vi "Autonomous Independent.vi"() -> ()   [LabVIEW 2012]
doc: "This VI is called when autonomous begins, and will automatically be terminated when autonomous ends. You can carry out timed or sensor driven robot movement independently without needing to return to the caller."
uses:
  Robot Global Data.vi
  <vilib>/Rock Robotics/WPI/RobotDrive/WPI_RobotDriveArcadeDrive_Standard(NoSaturation).vi
panel:
  out "Shooter Tolerance":dbl
  out "Mode":u32
  out "Auton Mode":bool[](array[boolean])
  in  "Blank 2":i32=7
  in  "Blank 1":i32
  out "Driver Station":bool[](array[boolean])
  out "Auton RPM Used":dbl
  out "Auton Pitch Used":dbl
  in  "Auton RPM 2":dbl=4200.0
  in  "Auton Pitch 2":dbl=29.5
  out "Analog 1 (V)":dbl
  out "Autonomous Modes":T1(ring)
  out "Current Movement, for debugging":T2 {"Y Joystick Value" scale=1.0..-1.0; "X Joystick Value" scale=-1.0..1.0}
  in  "Array of robot movements":T3(array[cluster]) {"Y Joystick Value" scale=1.0..-1.0; "X Joystick Value" scale=-1.0..1.0}
  # "Palmetto: Auton RPM was 4200, Pitch was 29.5"
  # "WING"
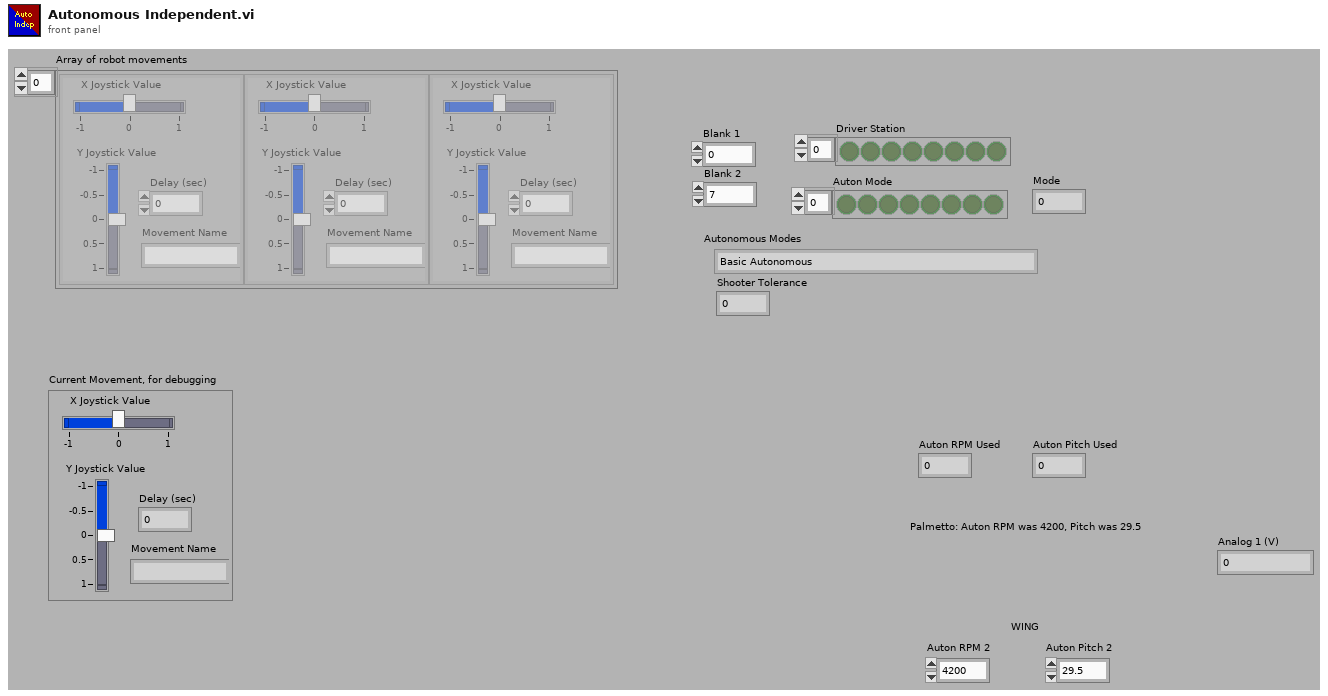
[diagram p1: front panel]
types:
  T1 = enum16{"Basic Autonomous", "Delayed Autonomous", "Shoot and Line Up With Protected Feeder Station", "Shoot and Line Up With Unprotected Feeder Station"}
  T2 = cluster{"X Joystick Value":dbl, "Y Joystick Value":dbl, "Delay (sec)":dbl, "Movement Name":string}
  T3 = cluster{"X Joystick Value":dbl, "Y Joystick Value":dbl, "Delay (sec)":dbl, "Movement Name":string}[]
  T4 = typedef "WPI_JoystickDevRef.ctl" = cluster{"Device":T5}
  T5 = typedef "WPI_JoystickDeviceEnum.ctl" = enum16{"USB 1", "USB 2", "USB 3", "USB 4", "Kinect 1", "Kinect 2"}
  T6 = cluster{"axis 1 (x)":dbl, "axis 2 (y)":dbl, "axis 3 (throttle)":dbl, "axis 4":dbl, "axis 5":dbl, "axis 6":dbl}
  T7 = typedef "WPI_RobotDriveDevRef.ctl" = cluster{"DevStatus":errorcluster, "Motors[]":T8[], "Square Inputs":bool, "Max Output":dbl, "Isochronous":bool}
  T8 = typedef "WPI_MotorControlDeviceRef.ctl" = cluster{"DeviceStatus":errorcluster, "Type":enum16{"PWM", "CAN"}, "PWM":cluster{"Digital Module":T9, "PWM Channel":T10, "DeadBand":T11}, "CAN":cluster{"Device Number":u8, "Control Mode":T12, "Semaphore":T13, "Max Vout":dbl}, "Invert":bool, "TransformRef":T14, "InvTransformRef":T14}
  T9 = typedef "FPGA_TypedefDigitalModule.ctl" = enum16{"Digital Module 1", "Digital Module 2"}
  T10 = typedef "FPGA_DIOPWMChannel.ctl" = enum8{"PWM 1", "PWM 2", "PWM 3", "PWM 4", "PWM 5", "PWM 6", "PWM 7", "PWM 8", "PWM 9", "PWM 10", "Invalid"}
  T11 = typedef "WPI_PWMDeadband.ctl" = cluster{"Name":string, "maxPositivePwm":i32, "minPositivePwm":i32, "centerPwm":i32, "maxNegativePwm":i32, "minNegativePwm":i32, "angularRange":u16}
  T12 = typedef "WPI_CANJaguar_ControlMode.ctl" = enum8{"Percent VBus", "Current", "Speed", "Position", "Voltage"}
  T13 = typedef "Semaphore RefNum" = refnum<k1>
  T14 = typedef "WPI_PWMTransform_ConPane.ctl" = refnum<vi>
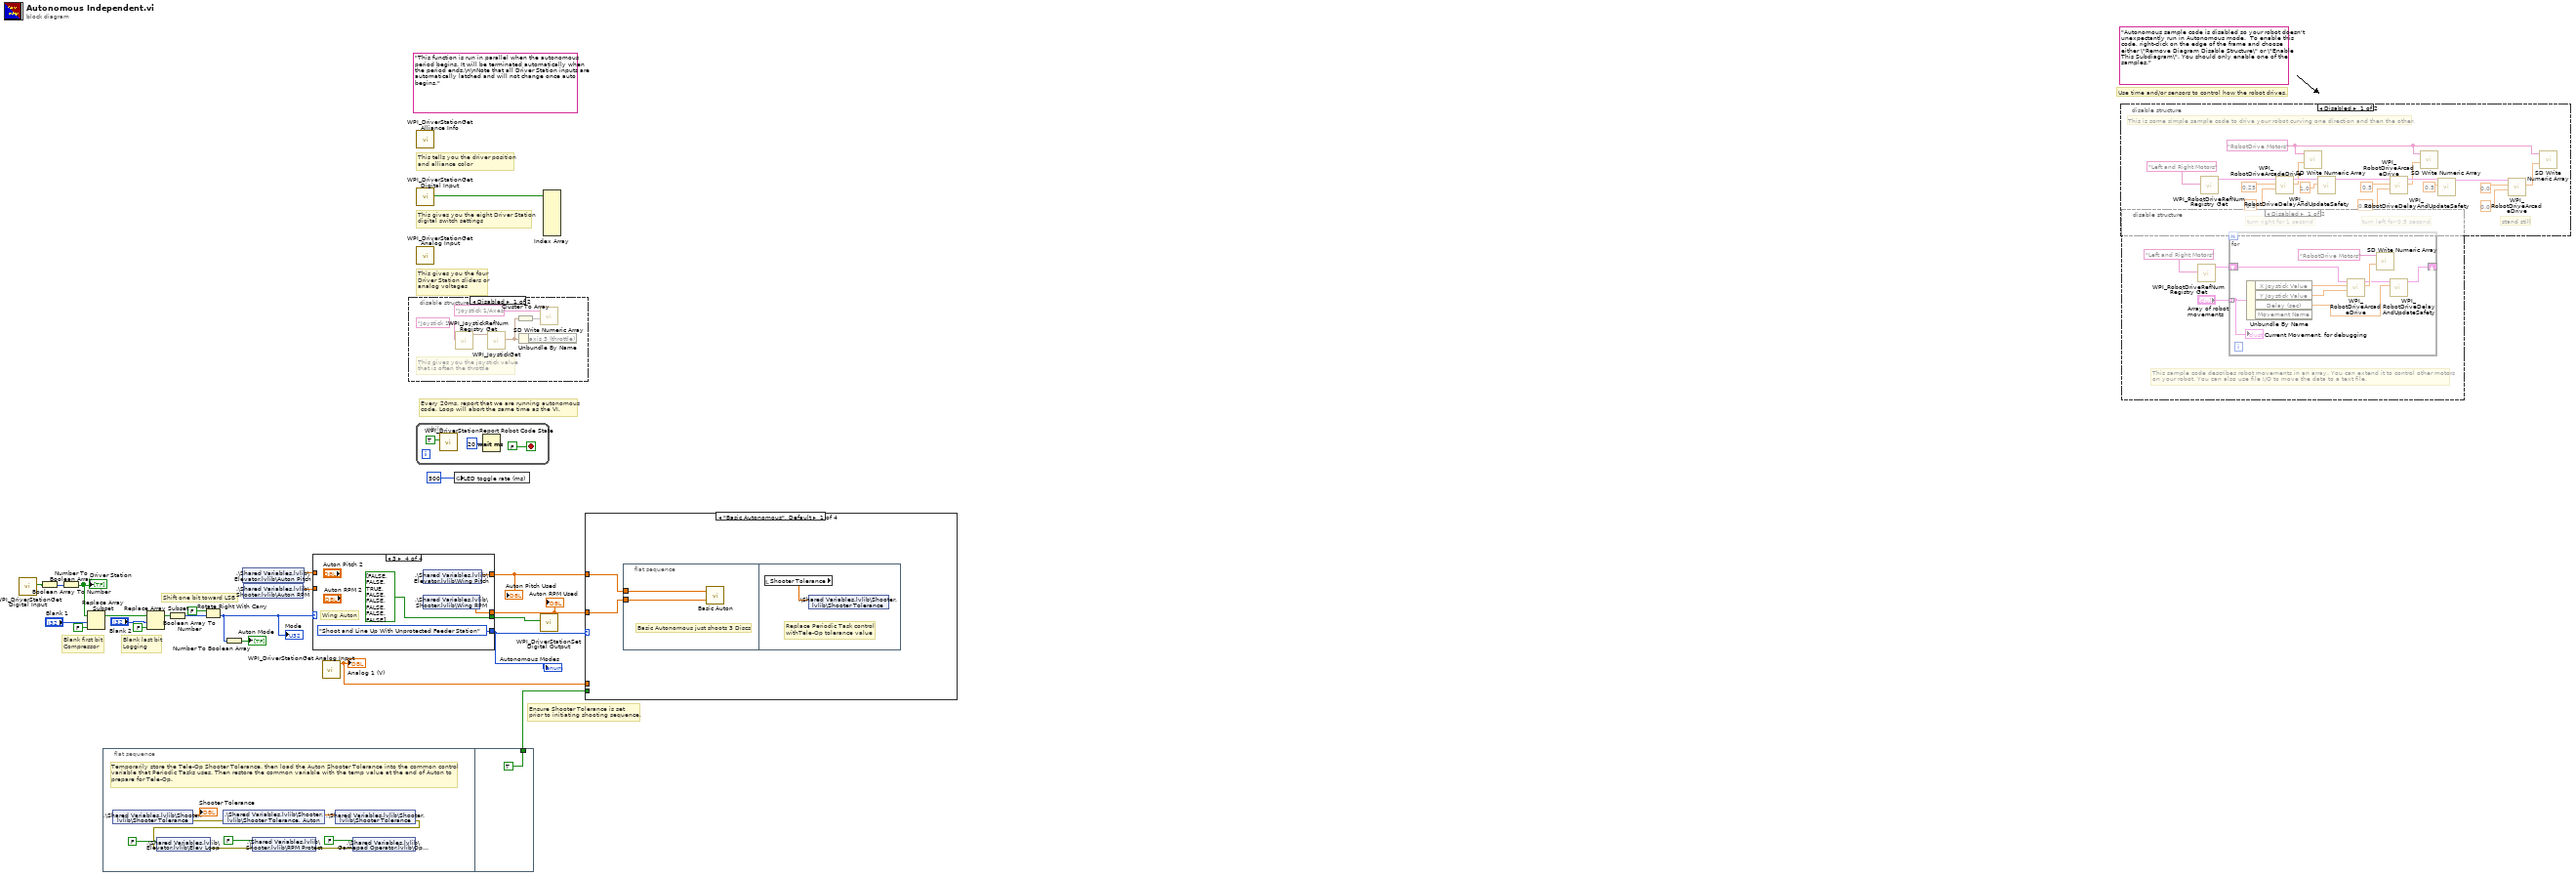
[diagram p0: block diagram]
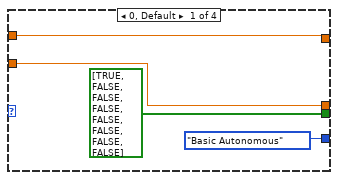
[diagram p3: hidden frame]
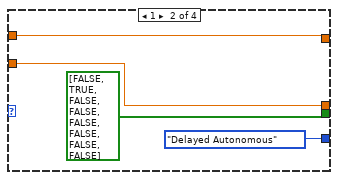
[diagram p4: hidden frame]
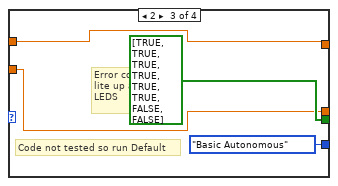
[diagram p5: hidden frame]
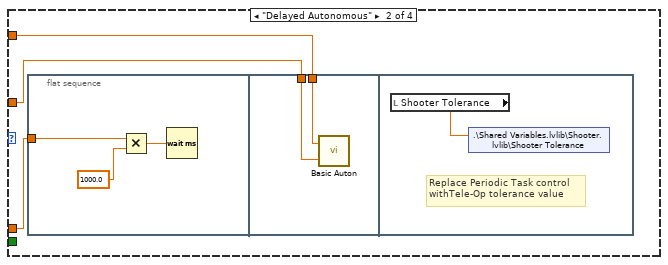
[diagram p6: hidden frame]
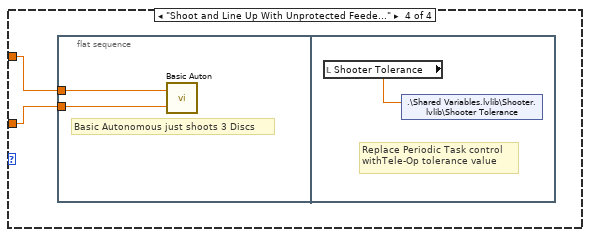
[diagram p8: hidden frame]
diagram:
  (unwired) "Autonomous sample code is disabled so your robot doesn't unexpectantly run in Autonomous mode.  To enable this code, right-click on the edge of the frame and choose either \"Remove Diagram Disable Structure\" or \"Enable This Subdiagram\". You should only enable one of the samples."
  (unwired) "This function is run in parallel when the autonomous period begins. It will be terminated automatically when the period ends.\n\nNote that all Driver Station inputs are automatically latched and will not change once auto begins."
  # "Ensure Shooter Tolerance is set\nprior to initiating shooting sequence."
  # "Shift one bit toward LSB"
  # "Blank last bit\nLogging"
  # "Blank first bit\nCompressor"
  # "Every 20ms, report that we are running autonomous\ncode. Loop will abort the same time as the VI."
  # "Use time and/or sensors to control how the robot drives."
  # "This tells you the driver position\nand alliance color"
  # "This gives you the eight Driver Station\ndigital switch settings"
  # "This gives you the four\nDriver Station sliders or\nanalog voltages"
  n1 = call <vilib>:"WPI_DriverStationGet Digital Input.vi"() -> ("Driver Station Digital Input (1-8)"=w19:bool[])  [unwired: 11 in]
  n2 = Boolean Array To Number(Boolean array=w19) -> (number=w5:u32)
  n3 = Number To Boolean Array(number=w5) -> (Boolean array=w15:bool[])
  "Driver Station" <- w15
  n4 = Replace Array Subset(array=w15, new element=FALSE ("new element/subarray"), index="Blank 1") -> (w10:bool[])
  n5 = flat-sequence {
    tunnel: [TRUE] -> w1
    frame #0 {
      # "Temporarily store the Tele-Op Shooter Tolerance, then load the Auton Shooter Tolerance into the common control \nvariable that Periodic Tasks uses. Then restore the common variable with the temp value at the end of Auton to \nprepare for Tele-Op."
      n6 = shared-variable ".\\Shared Variables.lvlib\\Shooter.lvlib\\Shooter Tolerance"() -> (→"Shooter Tolerance":dbl, error out=w27:errorcluster)  [unwired: 1 in]
      n7 = shared-variable ".\\Shared Variables.lvlib\\Shooter.lvlib\\Shooter Tolerance, Auton"(error in=w27) -> (w29:dbl)  [unwired: 1 out]
      n8 = shared-variable ".\\Shared Variables.lvlib\\Shooter.lvlib\\Shooter Tolerance"(w29) -> (error out=w26:errorcluster)  [unwired: 1 in]
      n9 = shared-variable ".\\Shared Variables.lvlib\\Elevator.lvlib\\Elev Loop"(FALSE ("ElevLoop"), error in=w26) -> (error out=w25:errorcluster)
      n10 = shared-variable ".\\Shared Variables.lvlib\\Shooter.lvlib\\RPM Protect"(FALSE ("collector_override"), error in=w25) -> (error out=w24:errorcluster)
      n11 = shared-variable ".\\Shared Variables.lvlib\\Gamepad Operator.lvlib\\Op Button 4"(FALSE ("Loading"), error in=w24) -> ()  [unwired: 1 out]
    }
    frame #1 {
    }
  }
  n12 = Replace Array Subset(array=w10, new element=FALSE ("new element/subarray"), index="Blank 2") -> (w9:bool[])
  n13 = Boolean Array To Number(Boolean array=w9) -> (number=w7:u32)
  n14 = Rotate Right With Carry(2:w7, 3:FALSE ("carry")) -> (0:w4:u32)  [unwired: 1 out]
  "Mode" <- w4
  n15 = Number To Boolean Array(number=w4) -> (Boolean array=→"Auton Mode":bool[])
  n16 = shared-variable ".\\Shared Variables.lvlib\\Elevator.lvlib\\Auton Pitch"() -> (w2:dbl)  [unwired: 1 in, 1 out]
  n17 = shared-variable ".\\Shared Variables.lvlib\\Shooter.lvlib\\Auton RPM"() -> (w3:dbl)  [unwired: 1 in, 1 out]
  n18 = case shown="3" w4 {
    tunnel: [T1."Basic Autonomous" ("Autonomous Modes") T1."Delayed Autonomous" ("Autonomous Modes") T1."Basic Autonomous" ("Autonomous Modes") T1."Shoot and Line Up With Unprotected Feeder Station" ("Autonomous Modes")] -> w21
    tunnel: [bool[] [TRUE, FALSE, FALSE, FALSE, FALSE, FALSE, FALSE, FALSE] ("Driver Station Digital Output (1-8)") bool[] [FALSE, TRUE, FALSE, FALSE, FALSE, FALSE, FALSE, FALSE] ("Driver Station Digital Output (1-8)") bool[] [TRUE, TRUE, TRUE, TRUE, TRUE, TRUE, FALSE, FALSE] ("Driver Station Digital Output (1-8)") bool[] [FALSE, FALSE, TRUE, FALSE, FALSE, FALSE, FALSE, FALSE] ("Driver Station Digital Output (1-8)")] -> w18
    tunnel: [w35 w39 w43 w47] -> w17
    tunnel: [w34 w38 w42 w46] -> w16
    tunnel: w2 -> [w35 w39 w43 _]
    tunnel: w3 -> [w34 w38 w42 _]
    frame 0, Default {
    }
    frame 1 {
    }
    frame 2 {
      # "Error cond\nlite up all\nLEDS"
      # "Code not tested so run Default"
    }
    frame 3 {
      # "Wing Auton"
      n19 = shared-variable ".\\Shared Variables.lvlib\\Elevator.lvlib\\Wing Pitch"() -> (w47:dbl)  [unwired: 1 in, 1 out]
      n20 = shared-variable ".\\Shared Variables.lvlib\\Shooter.lvlib\\Wing RPM"() -> (w46:dbl)  [unwired: 1 in, 1 out]
    }
  }
  "Autonomous Modes" <- w21
  "Auton Pitch Used" <- w17
  "Auton RPM Used" <- w16
  n21 = call <vilib>:"WPI_DriverStationGet Analog Input.vi"() -> ("Analog 1 (V)"=w20:dbl)  [unwired: 8 in, 3 out]
  "Analog 1 (V)" <- w20
  n22 = disable-structure shown="Disabled" {
    frame Disabled {
      # "This gives you the joystick value\nthat is often the throttle"
      n23 = call <vilib>:"WPI_JoystickRefNum Registry Get.vi"("refnum name"="Joystick 1") -> ("JoystickDevRef"=w53:T4)  [unwired: 1 in, 9 out]
      n24 = call <vilib>:"WPI_JoystickGet.vi"("JoystickDevRef"=w53) -> ("Axes"=w51:T6)  [unwired: 1 in, 5 out]
      n25 = Cluster To Array(cluster=w51) -> (array=w52:dbl[])
      n26 = Unbundle By Name(w51) -> ()  [unwired: 1 out]
      n27 = call <vilib>:"SD Write Numeric Array.vi"("Numeric Array"=w52, "Name"="Joystick 1/Axes") -> ()  [unwired: 8 in, 2 out]
    }
    frame Enabled {
    }
  }
  n28 = while {
    stop <- FALSE stop-if-true
    n29 = call <vilib>:"WPI_DriverStationReport Robot Code State.vi"("Autonomous"=TRUE) -> ()  [unwired: 10 in, 1 out]
    n30 = Wait (ms)(milliseconds to wait=u32 20) -> ()  [unwired: 1 out]
  }
  n31 = call <vilib>:"WPI_DriverStationGet Alliance Info.vi"() -> ()  [unwired: 12 out]
  n32 = call <vilib>:"WPI_DriverStationGet Digital Input.vi"() -> ("Driver Station Digital Input (1-8)"=w23:bool[])  [unwired: 11 out]
  n33 = call <vilib>:"WPI_DriverStationGet Analog Input.vi"() -> ()  [unwired: 12 out]
  n34 = global write "Robot Global Data.vi" "LED toggle rate (ms)"(u32 500 ("LED ms toggle rate")) -> ()
  n35 = call <vilib>:"WPI_DriverStationSet Digital Output.vi"("Driver Station Digital Output (1-8)"=w18) -> ()  [unwired: 10 in, 1 out]
  n36 = Index Array(array=w23) -> ()  [unwired: 8 in, 8 out]
  n37 = case shown="\"Basic Autonomous\", Default" w21 {
    tunnel: w20 -> [_ w65 _ _]
    tunnel: w17 -> [w59 w64 _ w73]
    tunnel: w16 -> [w58 w63 _ w72]
    tunnel: w1 -> [_ _ _ _]
    frame "Basic Autonomous", Default {
      n38 = flat-sequence {
        tunnel: w59 -> [w61]
        tunnel: w58 -> [w60]
        frame #0 {
          # "Basic Autonomous just shoots 3 Discs"
          n39 = call "Basic Auton.vi"("Auton RPM"=w60, "Auton Pitch"=w61) -> ()  [unwired: 1 in]
        }
        frame #1 {
          # "Replace Periodic Task control\nwithTele-Op tolerance value"
          n40 = local read "Shooter Tolerance"() -> (w62:dbl)
          n41 = shared-variable ".\\Shared Variables.lvlib\\Shooter.lvlib\\Shooter Tolerance"(w62) -> ()  [unwired: 1 in, 1 out]
        }
      }
    }
    frame "Delayed Autonomous" {
      n42 = flat-sequence {
        tunnel: w65 -> [w66]
        tunnel: w64 -> [w70]
        tunnel: w63 -> [w69]
        frame #0 {
          n43 = Multiply(x=w66, y=1000.0) -> (x*y=w68:dbl)
          n44 = Wait (ms)(milliseconds to wait=w68) -> ()  [unwired: 1 out]
        }
        frame #1 {
          n45 = call "Basic Auton.vi"("Auton RPM"=w69, "Auton Pitch"=w70) -> ()  [unwired: 1 in]
        }
        frame #2 {
          # "Replace Periodic Task control\nwithTele-Op tolerance value"
          n46 = local read "Shooter Tolerance"() -> (w71:dbl)
          n47 = shared-variable ".\\Shared Variables.lvlib\\Shooter.lvlib\\Shooter Tolerance"(w71) -> ()  [unwired: 1 in, 1 out]
        }
      }
    }
    frame "Shoot and Line Up With Protected Feeder Station" {
    }
    frame "Shoot and Line Up With Unprotected Feeder Station" {
      n48 = flat-sequence {
        tunnel: w73 -> [w75]
        tunnel: w72 -> [w74]
        frame #0 {
          # "Basic Autonomous just shoots 3 Discs"
          n49 = call "Basic Auton.vi"("Auton RPM"=w74, "Auton Pitch"=w75) -> ()  [unwired: 1 in]
        }
        frame #1 {
          # "Replace Periodic Task control\nwithTele-Op tolerance value"
          n50 = local read "Shooter Tolerance"() -> (w76:dbl)
          n51 = shared-variable ".\\Shared Variables.lvlib\\Shooter.lvlib\\Shooter Tolerance"(w76) -> ()  [unwired: 1 in, 1 out]
        }
      }
    }
  }
  n52 = disable-structure shown="Disabled" {
    frame Disabled {
      w77 = "RobotDrive Motors" ("Name")
      # "This is some simple sample code to drive your robot curving one direction and then the other."
      # "stand still"
      # "turn left for 0.5 second"
      # "turn right for 1 second"
      n53 = call <vilib>:"WPI_RobotDriveRefNum Registry Get.vi"("refnum name"="Left and Right Motors") -> ("RobotDriveDevRef"=w81:T7)  [unwired: 1 in, 9 out]
      n54 = call-poly <vilib>:"WPI_RobotDriveArcadeDrive.vi"("Y axis value"=0.5 ("X axis value"), "X axis value"=0.25, "RobotDriveDevRef"=w81) -> ("Motor Values"=w80:dbl[], "RobotDriveDevRef"=w88:T7)  [unwired: 1 in, 6 out]
      n55 = call <vilib>:"SD Write Numeric Array.vi"("Numeric Array"=w80, "Name"=w77) -> ()  [unwired: 8 in, 2 out]
      n56 = call <vilib>:"WPI_RobotDriveDelayAndUpdateSafety.vi"("Delay (s)"=1.0, "RobotDriveDevRef"=w88) -> ("RobotDriveDevRef 2"=w87:T7)  [unwired: 8 in, 1 out]
      n57 = call-poly <vilib>:"WPI_RobotDriveArcadeDrive.vi"("Y axis value"=0.25 ("X axis value"), "X axis value"=0.5, "RobotDriveDevRef"=w87) -> ("Motor Values"=w79:dbl[], "RobotDriveDevRef"=w86:T7)  [unwired: 1 in, 6 out]
      n58 = call <vilib>:"SD Write Numeric Array.vi"("Numeric Array"=w79, "Name"=w77) -> ()  [unwired: 8 in, 2 out]
      n59 = call <vilib>:"WPI_RobotDriveDelayAndUpdateSafety.vi"("Delay (s)"=0.5, "RobotDriveDevRef"=w86) -> ("RobotDriveDevRef 2"=w85:T7)  [unwired: 8 in, 1 out]
      n60 = call-poly <vilib>:"WPI_RobotDriveArcadeDrive.vi"("Y axis value"=0.0 ("X axis value"), "X axis value"=0.0, "RobotDriveDevRef"=w85) -> ("Motor Values"=w78:dbl[])  [unwired: 1 in, 7 out]
      n61 = call <vilib>:"SD Write Numeric Array.vi"("Numeric Array"=w78, "Name"=w77) -> ()  [unwired: 8 in, 2 out]
    }
    frame Enabled {
    }
  }
  n62 = disable-structure shown="Disabled" {
    frame Disabled {
      # "This sample code describes robot movements in an array. You can extend it to control other motors\non your robot. You can also use file I/O to move the data to a text file."
      n63 = call <vilib>:"WPI_RobotDriveRefNum Registry Get.vi"("refnum name"="Left and Right Motors") -> ("RobotDriveDevRef"=w96:T7)  [unwired: 1 in, 9 out]
      n64 = for {
        shift-right: [w102] -> _
        shift-left: w96 -> [w103]
        tunnel: "Array of robot movements" -> [w98] mode=indexing
        n65 = Unbundle By Name(w98) -> ("X Joystick Value"=w101:dbl, "Y Joystick Value"=w100:dbl, "Delay (sec)"=w99:dbl)  [unwired: 1 out]
        n66 = call-poly <vilib>:"WPI_RobotDriveArcadeDrive.vi"("Y axis value"=w100, "X axis value"=w101, "RobotDriveDevRef"=w103) -> ("Motor Values"=w105:dbl[], "RobotDriveDevRef"=w104:T7)  [unwired: 1 in, 6 out]
        n67 = call <vilib>:"SD Write Numeric Array.vi"("Numeric Array"=w105, "Name"="RobotDrive Motors") -> ()  [unwired: 8 in, 2 out]
        n68 = call <vilib>:"WPI_RobotDriveDelayAndUpdateSafety.vi"("Delay (s)"=w99, "RobotDriveDevRef"=w104) -> ("RobotDriveDevRef 2"=w102:T7)  [unwired: 8 in, 1 out]
        "Current Movement, for debugging" <- w98
      }
    }
    frame Enabled {
    }
  }
